vi "AOICoords.vi"(0 "X-Y data":cluster{"x coord":dbl[], "y coord":dbl[]} {"y coord" format="%.2f"; "x coord" format="%.2f"}) -> (5 "start row for pts":i32[](array[numeric]), 6 "start column for pts":i32[](array[numeric]), 7 "# pts to take in row":i32[](array[numeric]))   [LabVIEW 2022 SP3]
uses:
  <vilib>/Analysis/NI_AALPro.lvlib
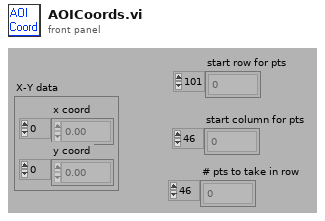
[diagram p1: front panel]
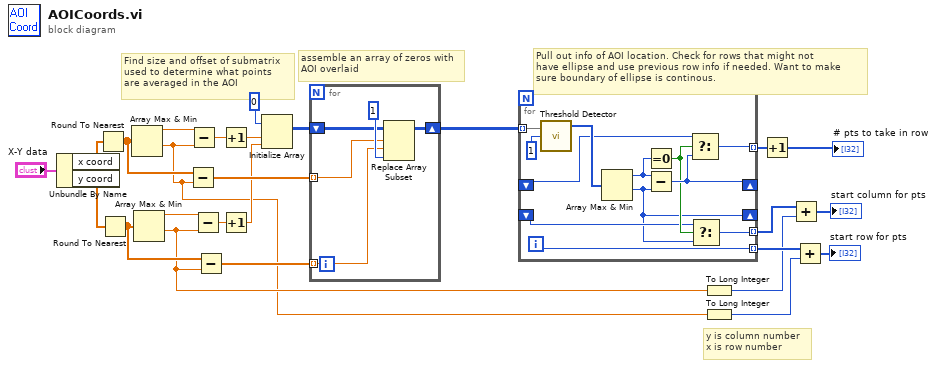
[diagram p0: block diagram]
diagram:
  # "Find size and offset of submatrix\nused to determine what points\nare averaged in the AOI"
  # "Pull out info of AOI location. Check for rows that might not\nhave ellipse and use previous row info if needed. Want to make\nsure boundary of ellipse is continous."
  # "y is column number\nx is row number"
  # "assemble an array of zeros with\nAOI overlaid"
  n1 = Unbundle By Name("X-Y data") -> ("x coord"=w18:dbl[], "y coord"=w20:dbl[])
  n2 = Round To Nearest(number=w18) -> (nearest integer value=w17:dbl[])
  n3 = Round To Nearest(number=w20) -> (nearest integer value=w19:dbl[])
  n4 = Array Max & Min(array=w17) -> (max value=w25:dbl, min value=w1:dbl)  [unwired: 2 out]
  n5 = Array Max & Min(array=w19) -> (max value=w24:dbl, min value=w2:dbl)  [unwired: 2 out]
  n6 = Subtract(x=w17, y=w1) -> (x-y=w15:dbl[])
  n7 = Subtract(x=w25, y=w1) -> (x-y=w23:dbl)
  n8 = Subtract(x=w24, y=w2) -> (x-y=w22:dbl)
  n9 = Subtract(x=w19, y=w2) -> (x-y=w14:dbl[])
  n10 = Increment(x=w23) -> (x+1=w8:dbl)
  n11 = Increment(x=w22) -> (x+1=w13:dbl)
  n12 = Initialize Array(i8 0, w8, w13) -> (w16:i8[][])
  n13 = for {
    shift-right: [w27] -> w11
    shift-left: w16 -> [w28]
    tunnel: w15 -> [w30] mode=indexing
    tunnel: w14 -> [w29] mode=indexing
    n14 = Replace Array Subset(array=w28, new element=i8 1, index (row)=w30, index (col)=w29) -> (w27:i8[][])
  }
  n15 = for {
    tunnel: w11 -> [w43] mode=indexing
    shift-right: [w39] -> _
    shift-left: _ -> [w38]
    tunnel: [w37] -> w12 mode=indexing
    shift-right: [w34] -> _
    shift-left: _ -> [w35]
    tunnel: [w33] -> w10 mode=indexing
    tunnel: [w32] -> w9 mode=indexing
    i -> [w32]
    n16 = call <vilib>:"Threshold Detector.vi"("threshold"=i8 1, "X"=w43) -> ("Indices"=w41:i32[])  [unwired: 1 in, 2 out]
    n17 = Array Max & Min(array=w41) -> (max value=w40:i32, min value=w34:i32)  [unwired: 2 out]
    n18 = Equal To 0?(x=w40) -> (x = 0?=w36:bool)
    n19 = Subtract(x=w40, y=w34) -> (x-y=w39:i32)
    n20 = Select(t=w38, s=w36, f=w39) -> (s? t:f=w37:i32)
    n21 = Select(t=w35, s=w36, f=w34) -> (s? t:f=w33:i32)
  }
  n22 = To Long Integer(number=w2) -> (32bit integer=w5:i32)
  n23 = To Long Integer(number=w1) -> (32bit integer=w4:i32)
  n24 = Increment(x=w12) -> (x+1=→"# pts to take in row":i32[])
  n25 = Add(x=w10, y=w5) -> (x+y=→"start column for pts":i32[])
  n26 = Add(x=w9, y=w4) -> (x+y=→"start row for pts":i32[])
